vi "NR_LSChannel.vi"(0 "appended path":path, 1 "deremapdata":cxt[][](array[numeric]), 2 "TransformPrcode_en":dbl, 3 "cellid":dbl, 4 "beltaDMRS":dbl, 5 "Nsym_slot":dbl, 6 "nslotnum":dbl, 7 "Second_DMRS_L":dbl, 8 "UL_DMRS_Config_type":dbl, 9 "prb_num":dbl, 10 "Frist_DMRS_L0":dbl, 11 "EN_CHES":dbl, 12 "DMRS_symbol":dbl, 13 "error in (no error)":errorcluster caption="错误输入（无错误）") -> (14 "equdata":cdb[](array[numeric]), 17 "slotlschanneldata":cdb[][](array[numeric]), 19 "error IO":errorcluster)   [LabVIEW 2015]
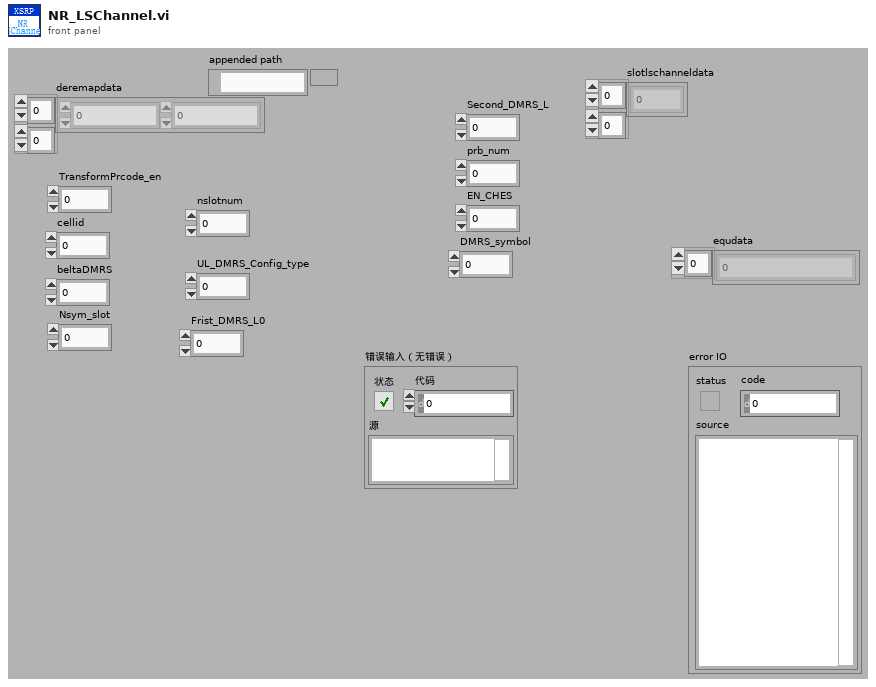
[diagram p1: front panel]
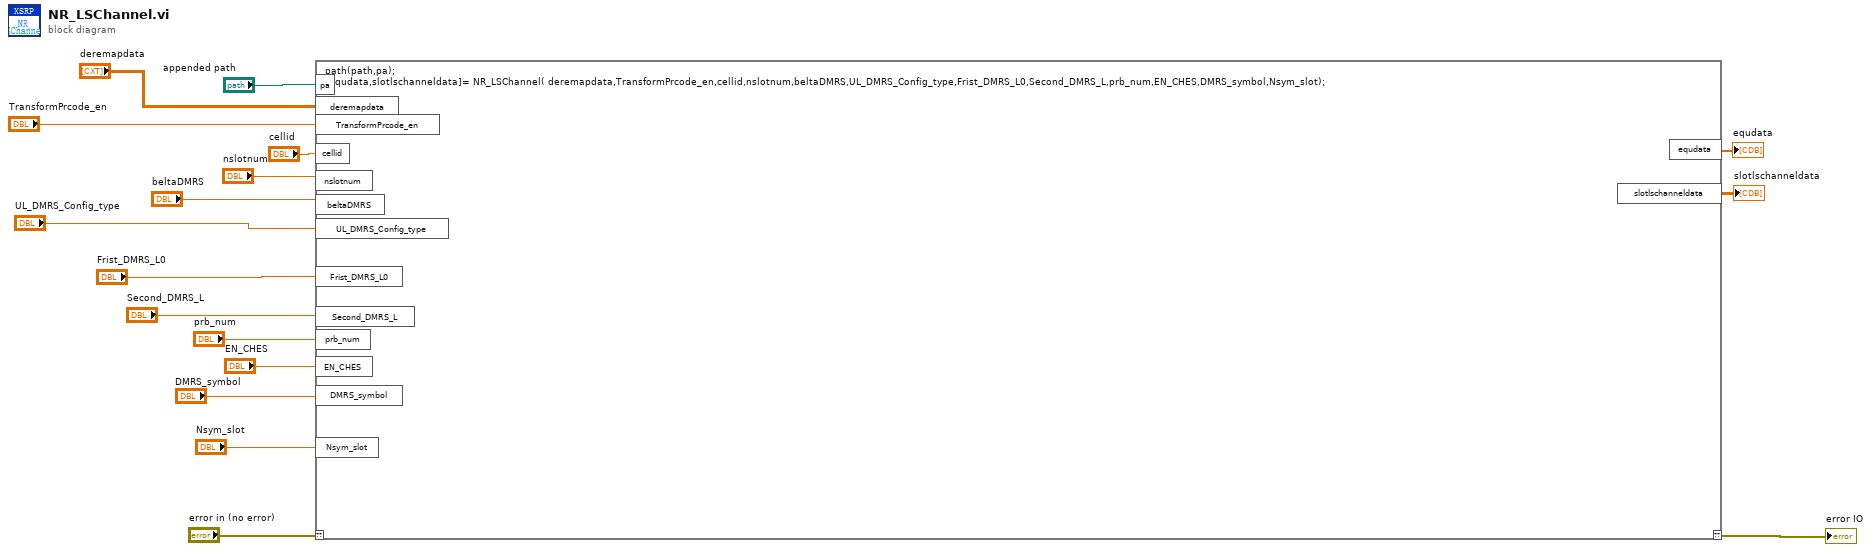
[diagram p0: block diagram]
diagram:
  n1 = script code="path(path,pa);\n[equdata,slotlschanneldata]= NR_LSChannel( deremapdata,TransformPrcode_en,cellid,nslotnum,beltaDMRS,UL_DMRS_Config_type,Frist_DMRS_L0,Second_DMRS_L,prb_num,EN_CHES,DMRS_symbol,Nsym_slot);"("??"="error in (no error)", "pa"="appended path", "deremapdata"="deremapdata", "TransformPrcode_en"="TransformPrcode_en", "cellid"="cellid", "nslotnum"="nslotnum", "beltaDMRS"="beltaDMRS", "UL_DMRS_Config_type"="UL_DMRS_Config_type", "Frist_DMRS_L0"="Frist_DMRS_L0", "Second_DMRS_L"="Second_DMRS_L", "prb_num"="prb_num", "EN_CHES"="EN_CHES", "DMRS_symbol"="DMRS_symbol", "Nsym_slot"="Nsym_slot") -> ("??"=→"error IO":errorcluster, "equdata"=→"equdata":cdb[], "slotlschanneldata"=→"slotlschanneldata":cdb[][])
